vi "SECoP_dataModifyInteger.vi"(6 "Value":i64, 7 "Position":u32, 8 "error in (no error)":errorcluster, 9 "Index":u32, 10 "SECoP_data":T1 {"ptr64" format="%.0x"; "ptr32" format="%.0x"}, 11 "DLL path (in)":T2) -> (0 "error out":errorcluster, 3 "DLL path (out)":T2)   [LabVIEW 2023, in "SECoP.lvlib"]
doc: "Call <b>\"SECoP_dataModifyInteger.vi\"</b> to change the numeric value (integer of SECoP_dataPtr).\n\n<b>DLL path</b> input and output of cluster from \"SECoP-Initialize.vi\"\n<b>SECoP_dataPtr</b> data to access\n<b>Position</b> points to a virtual flattened entry of the data type\n<b>Index</b> zero based index into array type or 0 for single type\n<b>Value</b> new value"
uses:
  SECoP.lvlib
  SECoP-libraries.ctl
  SECoP-data.ctl
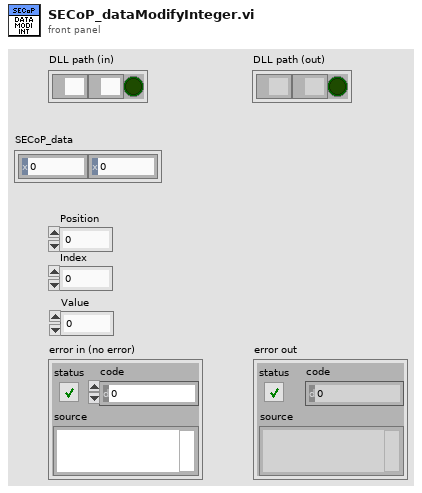
[diagram p1: front panel]
types:
  T1 = typedef "SECoP.lvlib/SECoP-data.ctl" = cluster{"ptr32":u32, "ptr64":u64}
  T2 = typedef "SECoP.lvlib/SECoP-libraries.ctl" = cluster{"serverDLL":path, "variantDLL":path, "cleanup_mode":bool}
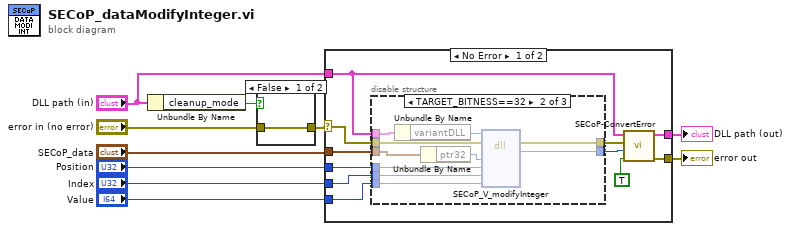
[diagram p0: block diagram]
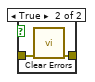
[diagram p2: hidden frame]
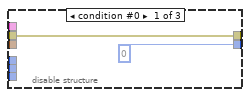
[diagram p3: hidden frame]
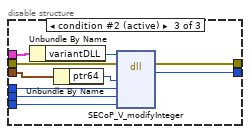
[diagram p4: hidden frame]
diagram:
  n1 = Unbundle By Name("DLL path (in)") -> ("cleanup_mode"=w8:bool)
  n2 = case shown="False" w8 {
    tunnel: "error in (no error)" -> [w11 w13]
    tunnel: [w11 w12] -> w6
    frame False {
    }
    frame True {
      n3 = call <vilib>:"Clear Errors.vi"("error in (no error)"=w13) -> ("error out"=w12:errorcluster)  [unwired: 5 in, 1 out]
    }
  }
  n4 = case shown="No Error" w6 {
    selector: w6 -> [w22 w47]
    tunnel: "DLL path (in)" -> [w16 w48]
    tunnel: [w23 w48] -> w10
    tunnel: [w24 w47] -> w9
    tunnel: "SECoP_data" -> [w17 _]
    tunnel: "Value" -> [w19 _]
    tunnel: "Position" -> [w15 _]
    tunnel: "Index" -> [w14 _]
    frame No Error {
      n5 = disable-structure shown="TARGET_BITNESS==32" {
        disable-tunnel: w22 -> [w26 w34 w46]
        disable-tunnel: w16 -> [_ w35 w45]
        disable-tunnel: [0 w32 w44] -> w21
        disable-tunnel: w19 -> [_ w33 w43]
        disable-tunnel: w15 -> [_ w28 w38]
        disable-tunnel: [w26 w36 w42] -> w18
        disable-tunnel: w17 -> [_ w30 w40]
        disable-tunnel: w14 -> [_ w27 w37]
        frame condition #0 {
        }
        frame condition #1 {
          n6 = Unbundle By Name(w35) -> ("variantDLL"=w29:path)
          n7 = Unbundle By Name(w30) -> ("ptr32"=w31:u32)
          n8 = dll-call lib="Z:/Praktische_Aufgaben/SECoP-LabVIEW2015/32bit/SECoP32.dll" fn="SECoP_V_modifyInteger"(path in=w29, error in=w34, "Data"=w31, "Position"=w28, "Index"=w27, "Value"=w33) -> (error out=w36:errorcluster, "return type"=w32:i32)  [unwired: 5 in, 1 out]
        }
        frame condition #2 (active) {
          n9 = Unbundle By Name(w45) -> ("variantDLL"=w39:path)
          n10 = Unbundle By Name(w40) -> ("ptr64"=w41:u64)
          n11 = dll-call lib="Z:/Praktische_Aufgaben/SECoP-LabVIEW2015/32bit/SECoP32.dll" fn="SECoP_V_modifyInteger"(path in=w39, error in=w46, "Data"=w41, "Position"=w38, "Index"=w37, "Value"=w43) -> (error out=w42:errorcluster, "return type"=w44:i32)  [unwired: 5 in, 1 out]
        }
      }
      n12 = call "SECoP-ConvertError.vi"("return is boolean"=TRUE, "return code"=w21, "error in (no error)"=w18, "DLL path (in)"=w16) -> ("error out"=w24:errorcluster, "DLL path (out)"=w23:T2)  [unwired: 6 in]
    }
    frame Error {
    }
  }
  "DLL path (out)" <- w10
  "error out" <- w9
